vi "PH_AWG-510.Evt Call Set Output Settings.vi"(0 "i ref in":refnum<vi>, 1 "Instance":string, 2 "Wanted Output Settings":T1={"Activate Channel"=FALSE, "VPP (V)"=0.0, "Clock (Hz)"=0.0, "File Name (Device)"="", "#1"=0, "#2"=0, "#3"=0, "#4"=0, "#5"=0, "#6"=0, "#7"=0, "#8"=0, "#9"=0, "#10"=0, "#11"=0, "#12"=0, "#13"=0, "#14"=0, "#15"=0, "#16"=0, "#17"=0, "#18"=0, "#19"=0, "#20"=0, "Offset (V)"=-1.0} {"#20" max=1023 step=1 scale=0.0..1023.0; "#19" max=1023 step=1 scale=0.0..1023.0; "#18" max=1023 step=1 scale=0.0..1023.0; "#17" max=1023 step=1 scale=0.0..1023.0; "#16" max=1023 step=1 scale=0.0..1023.0; "#15" max=1023 step=1 scale=0.0..1023.0; "#14" max=1023 step=1 scale=0.0..1023.0; "#13" max=1023 step=1 scale=0.0..1023.0; "#12" max=1023 step=1 scale=0.0..1023.0; "#11" max=1023 step=1 scale=0.0..1023.0; "#10" max=1023 step=1 scale=0.0..1023.0; "#9" max=1023 step=1 scale=0.0..1023.0; "#8" max=1023 step=1 scale=0.0..1023.0; "#7" max=1023 step=1 scale=0.0..1023.0; "#6" max=1023 step=1 scale=0.0..1023.0; "#5" max=1023 step=1 scale=0.0..1023.0; "#4" max=1023 step=1 scale=0.0..1023.0; "#3" max=1023 step=1 scale=0.0..1023.0; "#2" max=1023 step=1 scale=0.0..1023.0; "#1" max=1023 step=1 scale=0.0..1023.0}, 5 "error in":errorcluster) -> (14 "i ref out":refnum<vi>, 19 "error out":errorcluster)   [LabVIEW 2014, in "PH_AWG-510.lvlib"]
doc: "This VI calls a method by a simple call."
uses:
  PH_AWG-510.lvlib
  PH_AWG-510.Output Settings.ctl
  CSCore/CSSystem/CoreLib/CoreLib.short 2 byte array.vi
  CSCore/CSSystem/CoreLib/CoreLib.string 2 byte array.vi
  CSCore/CSSystem/CoreLib/CoreLib.double 2 byte array.vi
  CSCore/CSSystem/CoreLib/CoreLib.lvlib
  CSCore/BaseProcess/BaseProcess.lvlib
panel:
  # "Waveform Pattern"
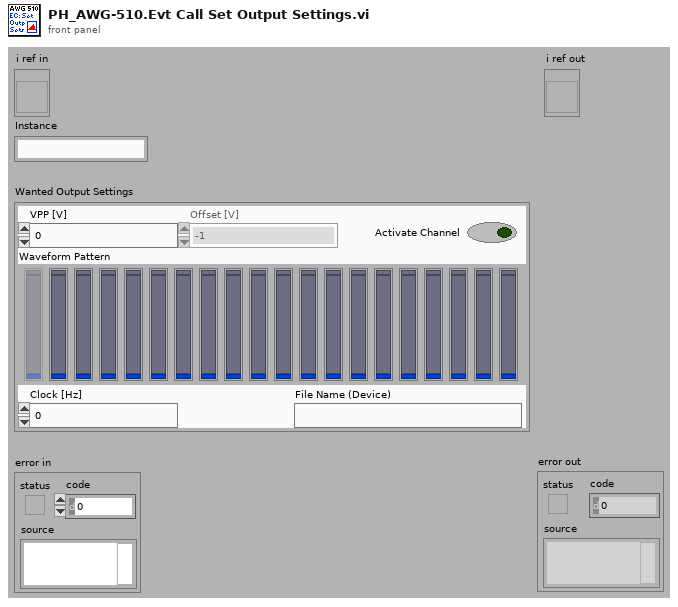
[diagram p1: front panel]
types:
  T1 = typedef "PH_AWG-510.lvlib/PH_AWG-510.Output Settings.ctl" = cluster{"Activate Channel":bool, "VPP (V)":dbl, "Clock (Hz)":dbl, "File Name (Device)":string, "#1":u16, "#2":u16, "#3":u16, "#4":u16, "#5":u16, "#6":u16, "#7":u16, "#8":u16, "#9":u16, "#10":u16, "#11":u16, "#12":u16, "#13":u16, "#14":u16, "#15":u16, "#16":u16, "#17":u16, "#18":u16, "#19":u16, "#20":u16, "Offset (V)":dbl}
  T2 = typedef "CoreDefs.rawDataType.ctl" = i8[]
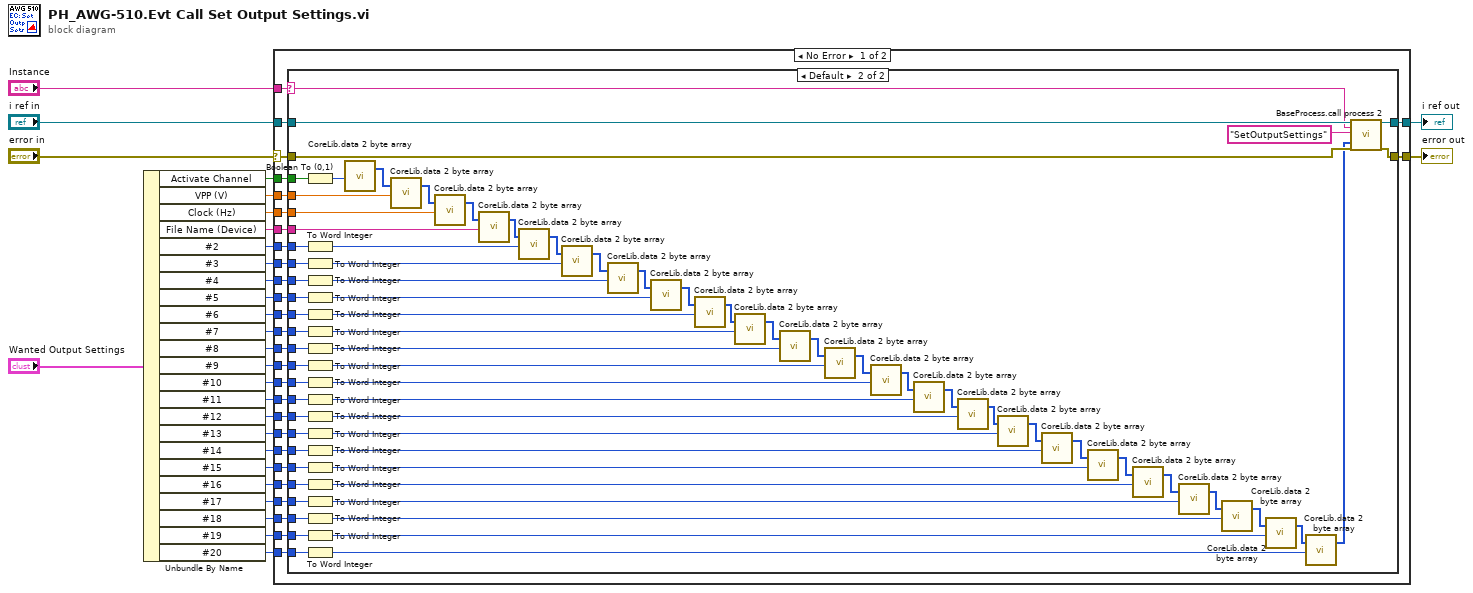
[diagram p0: block diagram]
diagram:
  n1 = Unbundle By Name("Wanted Output Settings") -> ("Activate Channel"=w23:bool, "VPP (V)"=w22:dbl, "Clock (Hz)"=w21:dbl, "File Name (Device)"=w20:string, "#2"=w19:u16, "#3"=w17:u16, "#4"=w16:u16, "#5"=w15:u16, "#6"=w14:u16, "#7"=w13:u16, "#8"=w12:u16, "#9"=w11:u16, "#10"=w10:u16, "#11"=w9:u16, "#12"=w8:u16, "#13"=w7:u16, "#14"=w6:u16, "#15"=w5:u16, "#16"=w4:u16, "#17"=w3:u16, "#18"=w2:u16, "#19"=w1:u16, "#20"=w18:u16)
  n2 = case shown="No Error" "error in" {
    selector: "error in" -> [w53 w132]
    tunnel: [w57 w132] -> w26
    tunnel: "Instance" -> [w52 _]
    tunnel: "i ref in" -> [w56 w133]
    tunnel: [w55 w133] -> w28
    tunnel: w23 -> [w54 _]
    tunnel: w22 -> [w51 _]
    tunnel: w21 -> [w50 _]
    tunnel: w20 -> [w49 _]
    tunnel: w19 -> [w48 _]
    tunnel: w18 -> [w47 _]
    tunnel: w17 -> [w46 _]
    tunnel: w16 -> [w45 _]
    tunnel: w15 -> [w44 _]
    tunnel: w14 -> [w43 _]
    tunnel: w13 -> [w42 _]
    tunnel: w12 -> [w41 _]
    tunnel: w11 -> [w40 _]
    tunnel: w10 -> [w39 _]
    tunnel: w9 -> [w38 _]
    tunnel: w8 -> [w37 _]
    tunnel: w7 -> [w36 _]
    tunnel: w6 -> [w35 _]
    tunnel: w5 -> [w34 _]
    tunnel: w4 -> [w33 _]
    tunnel: w3 -> [w32 _]
    tunnel: w2 -> [w31 _]
    tunnel: w1 -> [w30 _]
    frame No Error {
      n3 = case shown="Default" w52 {
        selector: w52 -> [_ w123]
        tunnel: [w59 w131] -> w57
        tunnel: w53 -> [w59 w129]
        tunnel: w56 -> [w58 w128]
        tunnel: [w58 w127] -> w55
        tunnel: w54 -> [_ w126]
        tunnel: w51 -> [_ w124]
        tunnel: w50 -> [_ w122]
        tunnel: w49 -> [_ w117]
        tunnel: w48 -> [_ w120]
        tunnel: w47 -> [_ w61]
        tunnel: w46 -> [_ w110]
        tunnel: w45 -> [_ w109]
        tunnel: w44 -> [_ w108]
        tunnel: w43 -> [_ w107]
        tunnel: w42 -> [_ w106]
        tunnel: w41 -> [_ w95]
        tunnel: w40 -> [_ w93]
        tunnel: w39 -> [_ w92]
        tunnel: w38 -> [_ w91]
        tunnel: w37 -> [_ w90]
        tunnel: w36 -> [_ w89]
        tunnel: w35 -> [_ w75]
        tunnel: w34 -> [_ w73]
        tunnel: w33 -> [_ w72]
        tunnel: w32 -> [_ w71]
        tunnel: w31 -> [_ w70]
        tunnel: w30 -> [_ w69]
        frame "", "N/A" {
        }
        frame Default {
          n4 = Boolean To (0,1)(Boolean=w126) -> (0, 1=w118:i16)
          n5 = To Word Integer(number=w120) -> (16bit integer=w116:i16)
          n6 = To Word Integer(number=w110) -> (16bit integer=w105:i16)
          n7 = To Word Integer(number=w109) -> (16bit integer=w104:i16)
          n8 = To Word Integer(number=w108) -> (16bit integer=w103:i16)
          n9 = To Word Integer(number=w107) -> (16bit integer=w102:i16)
          n10 = To Word Integer(number=w106) -> (16bit integer=w101:i16)
          n11 = To Word Integer(number=w95) -> (16bit integer=w88:i16)
          n12 = To Word Integer(number=w93) -> (16bit integer=w87:i16)
          n13 = To Word Integer(number=w92) -> (16bit integer=w86:i16)
          n14 = To Word Integer(number=w91) -> (16bit integer=w85:i16)
          n15 = To Word Integer(number=w90) -> (16bit integer=w84:i16)
          n16 = To Word Integer(number=w89) -> (16bit integer=w83:i16)
          n17 = To Word Integer(number=w75) -> (16bit integer=w67:i16)
          n18 = To Word Integer(number=w73) -> (16bit integer=w66:i16)
          n19 = To Word Integer(number=w72) -> (16bit integer=w65:i16)
          n20 = To Word Integer(number=w71) -> (16bit integer=w64:i16)
          n21 = To Word Integer(number=w70) -> (16bit integer=w63:i16)
          n22 = To Word Integer(number=w69) -> (16bit integer=w62:i16)
          n23 = To Word Integer(number=w61) -> (16bit integer=w60:i16)
          n24 = call-poly "CoreLib.data 2 byte array.vi"("i16"=w118) -> ("byteArray out"=w125:T2)  [unwired: 18 in]
          n25 = call-poly "CoreLib.data 2 byte array.vi"("byteArray"=w125, "f64"=w124) -> ("byteArray out"=w68:T2)  [unwired: 17 in]
          n26 = call-poly "CoreLib.data 2 byte array.vi"("byteArray"=w68, "f64"=w122) -> ("byteArray out"=w121:T2)  [unwired: 17 in]
          n27 = call-poly "CoreLib.data 2 byte array.vi"("byteArray"=w121, "string"=w117) -> ("byteArray out"=w119:T2)  [unwired: 17 in]
          n28 = call-poly "CoreLib.data 2 byte array.vi"("byteArray"=w119, "i16"=w116) -> ("byteArray out"=w111:T2)  [unwired: 17 in]
          n29 = call-poly "CoreLib.data 2 byte array.vi"("byteArray"=w111, "i16"=w105) -> ("byteArray out"=w115:T2)  [unwired: 17 in]
          n30 = call-poly "CoreLib.data 2 byte array.vi"("byteArray"=w115, "i16"=w104) -> ("byteArray out"=w114:T2)  [unwired: 17 in]
          n31 = call-poly "CoreLib.data 2 byte array.vi"("byteArray"=w114, "i16"=w103) -> ("byteArray out"=w113:T2)  [unwired: 17 in]
          n32 = call-poly "CoreLib.data 2 byte array.vi"("byteArray"=w113, "i16"=w102) -> ("byteArray out"=w112:T2)  [unwired: 17 in]
          n33 = call-poly "CoreLib.data 2 byte array.vi"("byteArray"=w112, "i16"=w101) -> ("byteArray out"=w94:T2)  [unwired: 17 in]
          n34 = call-poly "CoreLib.data 2 byte array.vi"("byteArray"=w94, "i16"=w88) -> ("byteArray out"=w96:T2)  [unwired: 17 in]
          n35 = call-poly "CoreLib.data 2 byte array.vi"("byteArray"=w96, "i16"=w87) -> ("byteArray out"=w100:T2)  [unwired: 17 in]
          n36 = call-poly "CoreLib.data 2 byte array.vi"("byteArray"=w100, "i16"=w86) -> ("byteArray out"=w99:T2)  [unwired: 17 in]
          n37 = call-poly "CoreLib.data 2 byte array.vi"("byteArray"=w99, "i16"=w85) -> ("byteArray out"=w98:T2)  [unwired: 17 in]
          n38 = call-poly "CoreLib.data 2 byte array.vi"("byteArray"=w98, "i16"=w84) -> ("byteArray out"=w97:T2)  [unwired: 17 in]
          n39 = call-poly "CoreLib.data 2 byte array.vi"("byteArray"=w97, "i16"=w83) -> ("byteArray out"=w76:T2)  [unwired: 17 in]
          n40 = call-poly "CoreLib.data 2 byte array.vi"("byteArray"=w76, "i16"=w67) -> ("byteArray out"=w77:T2)  [unwired: 17 in]
          n41 = call-poly "CoreLib.data 2 byte array.vi"("byteArray"=w77, "i16"=w66) -> ("byteArray out"=w78:T2)  [unwired: 17 in]
          n42 = call-poly "CoreLib.data 2 byte array.vi"("byteArray"=w78, "i16"=w65) -> ("byteArray out"=w82:T2)  [unwired: 17 in]
          n43 = call-poly "CoreLib.data 2 byte array.vi"("byteArray"=w82, "i16"=w64) -> ("byteArray out"=w81:T2)  [unwired: 17 in]
          n44 = call-poly "CoreLib.data 2 byte array.vi"("byteArray"=w81, "i16"=w63) -> ("byteArray out"=w80:T2)  [unwired: 17 in]
          n45 = call-poly "CoreLib.data 2 byte array.vi"("byteArray"=w80, "i16"=w62) -> ("byteArray out"=w79:T2)  [unwired: 17 in]
          n46 = call-poly "CoreLib.data 2 byte array.vi"("byteArray"=w79, "i16"=w60) -> ("byteArray out"=w74:T2)  [unwired: 17 in]
          n47 = call "BaseProcess.call process 2.vi"("i ref in"=w128, "Object"=w123, "Selector"="SetOutputSettings", "Data"=w74, "error in (no error)"=w129) -> ("i ref out"=w127:refnum<vi>, "error out"=w131:errorcluster)  [unwired: 13 in]
        }
      }
    }
    frame Error {
    }
  }
  "i ref out" <- w28
  "error out" <- w26
